vi "随机数.vi"() -> ()   [LabVIEW 2018]
panel:
  out "Numeric":dbl
  out "?":i16=1
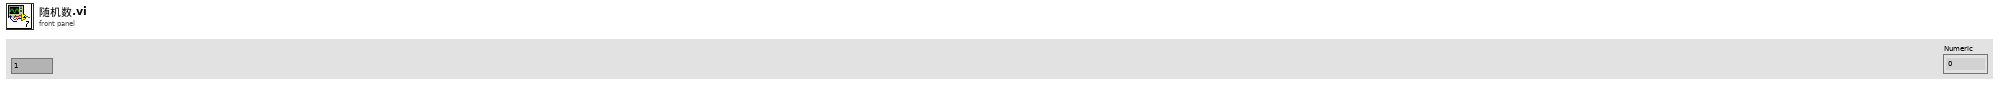
[diagram p1: front panel]
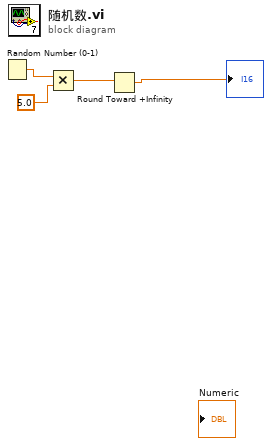
[diagram p0: block diagram]
diagram:
  n1 = Random Number (0-1)() -> (number: 0 to 1=w4:dbl)
  n2 = Multiply(x=w4, y=5.0) -> (x*y=w2:dbl)
  n3 = Round Toward +Infinity(x=w2) -> (ceil(x): smallest int >= x=→"?":dbl)
